vi "7.vi"   [LabVIEW 2020]
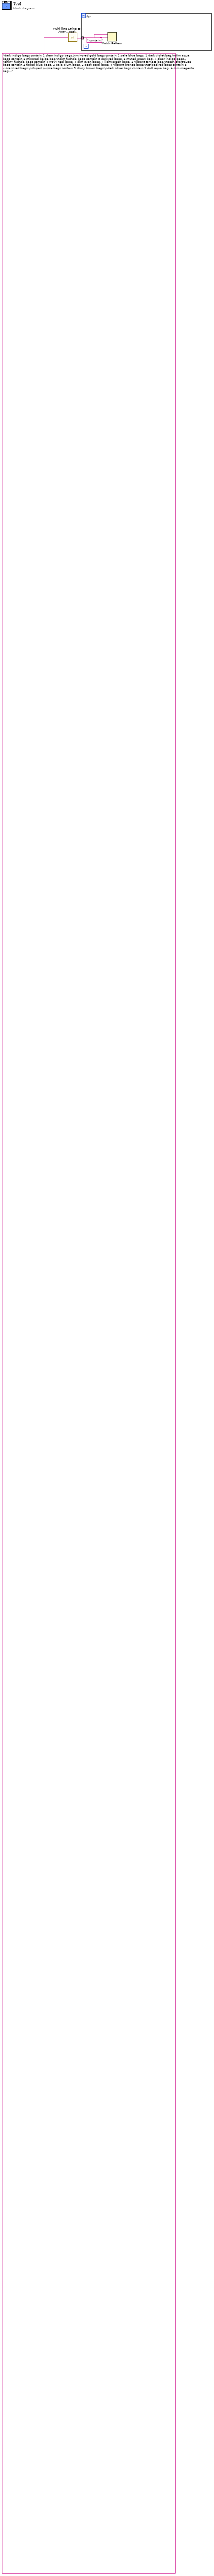
[diagram p0: block diagram]
diagram:
  n1 = call <userlib>:"Multi-line String to Array__ogtk.vi"("string"="dark indigo bags contain 2 clear indigo bags.\nmirrored gold bags contain 2 pale blue bags, 1 dark violet bag.\ndim aqua bags contain 1 mirrored beige bag.\ndim fuchsia bags contain 5 dark red bags, 1 muted green bag, 4 clear indigo bags.\nshiny fuchsia bags contain 4 wavy teal bags, 4 dim cyan bags, 4 light green bags, 1 vibrant tomato bag.\nposh chartreuse bags contain 2 faded blue bags, 2 pale plum bags, 2 posh coral bags, 4 vibrant bronze bags.\nstriped red bags contain 3 vibrant red bags.\nstriped purple bags contain 5 shiny brown bags.\ndark silver bags contain 1 dull aqua bag, 4 dim magenta bags.\ndark chartreuse bags contain 2 plaid black bags, 4 light bronze bags, 5 dotted cyan bags.\nshiny turquoise bags contain 1 shiny brown bag.\nshiny crimson bags contain no other bags.\nclear purple bags contain 4 bright red bags.\ndim white bags contain 4 posh violet bags, 2 light orange bags.\nplaid lime bags contain 4 muted silver bags, 2 vibrant tan bags.\nclear fuchsia bags contain 3 muted purple bags, 4 striped coral bags.\ndim plum bags contain 4 posh purple bags, 2 faded tomato bags, 1 mirrored magenta bag, 3 dull lime bags.\ndull white bags contain 4 light silver bags, 5 drab purple bags, 2 wavy orange bags, 1 striped coral bag.\ndull tomato bags contain 3 clear cyan bags, 5 dark turquoise bags, 4 light orange bags, 3 vibrant red bags.\nplaid tan bags contain 5 faded brown bags, 5 bright bronze bags.\nmirrored fuchsia bags contain 5 shiny brown bags, 3 dim magenta bags.\nwavy aqua bags contain 2 light beige bags, 3 vibrant white bags, 2 vibrant gold bags, 5 shiny tomato bags.\nclear white bags contain 3 dim maroon bags, 4 vibrant brown bags, 1 dim chartreuse bag.\nmuted yellow bags contain 3 shiny crimson bags, 4 posh purple bags, 2 dim plum bags, 3 shiny tomato bags.\nfaded cyan bags contain 5 mirrored crimson bags.\nposh violet bags contain 3 dim lavender bags, 3 vibrant teal bags.\nmirrored magenta bags contain 1 posh brown bag, 4 shiny teal bags, 2 shiny crimson bags.\nmirrored purple bags contain 2 clear aqua bags.\nwavy salmon bags contain 1 dull aqua bag, 1 dark silver bag.\nplaid purple bags contain 2 clear aqua bags, 5 pale brown bags, 3 bright chartreuse bags.\nposh teal bags contain 1 pale turquoise bag, 3 drab cyan bags.\npale tomato bags contain 2 dark beige bags.\nmuted plum bags contain 5 dotted gold bags, 5 shiny plum bags, 4 dull teal bags.\nwavy red bags contain 3 clear turquoise bags, 4 shiny chartreuse bags, 4 dotted maroon bags.\nwavy tomato bags contain 4 dark magenta bags, 1 faded bronze bag.\nshiny green bags contain 3 bright black bags, 2 clear turquoise bags.\nplaid turquoise bags contain 4 bright maroon bags.\nvibrant silver bags contain 5 bright chartreuse bags, 2 posh white bags, 3 drab tomato bags.\nposh olive bags contain 3 vibrant purple bags, 3 shiny crimson bags, 5 faded chartreuse bags.\nclear bronze bags contain 5 dark magenta bags.\nwavy teal bags contain 1 dim plum bag, 1 pale aqua bag, 2 posh purple bags, 2 pale orange bags.\nmuted beige bags contain 5 dotted brown bags, 4 mirrored green bags, 2 plaid blue bags.\nshiny maroon bags contain 2 pale green bags.\nwavy purple bags contain 5 dark bronze bags.\nvibrant cyan bags contain 2 drab blue bags, 5 pale brown bags, 1 mirrored magenta bag, 4 pale orange bags.\nwavy gray bags contain 5 pale crimson bags, 5 light aqua bags, 4 muted red bags.\nclear tomato bags contain 4 dark coral bags.\nshiny red bags contain 4 shiny tan bags, 4 pale cyan bags.\nmuted brown bags contain 5 dull olive bags, 2 pale silver bags, 5 faded plum bags.\nshiny violet bags contain 4 wavy teal bags.\nposh white bags contain 4 light fuchsia bags, 1 posh purple bag, 4 posh green bags.\ndim maroon bags contain 5 dim gold bags, 1 clear black bag.\ndull orange bags contain 1 clear teal bag, 3 dull gray bags.\nposh fuchsia bags contain 1 faded gold bag, 4 light bronze bags.\ndim bronze bags contain 1 bright fuchsia bag.\ndull salmon bags contain 5 muted tomato bags, 3 dull olive bags, 4 dark brown bags.\nposh yellow bags contain 5 dull indigo bags, 1 dotted green bag, 3 shiny chartreuse bags.\nmuted bronze bags contain 4 pale brown bags.\nwavy plum bags contain 4 shiny teal bags, 4 vibrant crimson bags.\ndark maroon bags contain 2 clear maroon bags, 3 light crimson bags.\nposh gray bags contain 2 drab maroon bags, 3 dotted aqua bags.\npale maroon bags contain 2 vibrant turquoise bags, 2 wavy tan bags, 5 clear orange bags, 2 clear beige bags.\nmirrored crimson bags contain 3 dark cyan bags, 3 dark silver bags.\nshiny bronze bags contain 3 drab tomato bags, 3 vibrant tan bags.\npale teal bags contain 4 clear brown bags, 4 vibrant gray bags, 3 bright plum bags, 4 dull olive bags.\nplaid maroon bags contain 1 mirrored blue bag, 4 bright chartreuse bags.\nplaid blue bags contain 4 light lime bags.\ndotted brown bags contain 5 shiny violet bags, 2 shiny lavender bags, 1 striped crimson bag.\npale purple bags contain 2 clear tomato bags, 5 vibrant orange bags, 5 dark green bags, 1 vibrant silver bag.\nclear lavender bags contain 1 wavy cyan bag, 5 dotted crimson bags, 5 dark bronze bags, 3 light bronze bags.\nlight cyan bags contain 5 light lime bags, 1 mirrored teal bag.\ndull blue bags contain 3 clear lime bags, 1 light turquoise bag, 1 shiny gray bag.\nfaded gray bags contain 2 faded crimson bags, 1 pale red bag, 3 striped bronze bags.\ndrab maroon bags contain 2 bright coral bags.\nplaid gold bags contain 2 shiny gold bags, 1 wavy fuchsia bag, 2 dull aqua bags, 4 mirrored indigo bags.\nmirrored orange bags contain 3 muted coral bags.\ndull yellow bags contain 1 drab maroon bag, 4 posh purple bags, 5 plaid cyan bags, 4 vibrant cyan bags.\nplaid aqua bags contain 2 bright silver bags, 2 posh blue bags, 3 drab olive bags, 2 mirrored fuchsia bags.\nshiny olive bags contain 3 dim tan bags, 1 dark gray bag, 4 mirrored brown bags, 5 mirrored magenta bags.\nwavy bronze bags contain 4 mirrored gray bags, 1 light lavender bag, 4 dull yellow bags.\ndotted orange bags contain 1 plaid teal bag, 5 pale silver bags, 1 drab bronze bag.\ndull magenta bags contain 1 muted violet bag, 2 muted black bags.\ndrab indigo bags contain 3 pale blue bags, 1 muted aqua bag, 3 bright fuchsia bags, 1 striped white bag.\nfaded turquoise bags contain 1 pale lavender bag, 1 shiny indigo bag.\nshiny lavender bags contain 2 faded bronze bags, 3 clear green bags, 5 dim turquoise bags, 5 striped olive bags.\nfaded yellow bags contain 1 faded chartreuse bag.\nvibrant gray bags contain 3 clear gold bags, 1 dotted coral bag, 4 light lime bags, 2 light lavender bags.\nbright aqua bags contain 2 faded chartreuse bags.\nbright yellow bags contain 4 dark blue bags.\nmirrored tomato bags contain 2 posh blue bags.\nshiny orange bags contain 3 striped black bags.\nbright tan bags contain 3 dim gold bags.\nlight fuchsia bags contain 4 dotted bronze bags, 2 posh purple bags.\nstriped coral bags contain 2 mirrored fuchsia bags, 4 faded chartreuse bags, 3 dull brown bags.\nbright cyan bags contain 3 mirrored lime bags, 2 posh purple bags, 3 light plum bags, 3 striped brown bags.\npale violet bags contain 3 wavy cyan bags.\nbright lavender bags contain 2 shiny crimson bags, 1 plaid magenta bag, 4 dark turquoise bags.\nwavy maroon bags contain 4 dull lavender bags, 2 dim turquoise bags, 2 light green bags, 1 clear lime bag.\ndrab tomato bags contain 1 light crimson bag, 5 faded gold bags, 5 drab cyan bags.\ndotted magenta bags contain 1 dotted beige bag.\nclear green bags contain 4 posh purple bags.\nshiny teal bags contain 2 pale turquoise bags.\nclear salmon bags contain 3 clear aqua bags.\ndark gold bags contain 1 pale tan bag.\nmirrored gray bags contain 1 muted purple bag.\nvibrant indigo bags contain 3 muted coral bags, 5 shiny gray bags, 1 dark yellow bag.\npale olive bags contain 2 posh white bags, 3 dull white bags, 5 light silver bags.\nbright bronze bags contain 3 dull yellow bags.\ndark yellow bags contain 1 bright black bag, 1 clear teal bag.\ndim cyan bags contain 4 wavy crimson bags, 4 muted green bags.\nshiny blue bags contain 1 pale beige bag, 1 plaid magenta bag, 1 dark magenta bag, 3 dim tomato bags.\npale green bags contain 5 dotted crimson bags, 5 posh purple bags, 4 pale aqua bags, 2 faded tomato bags.\nfaded coral bags contain 1 striped maroon bag, 5 drab salmon bags, 5 muted orange bags, 1 dark blue bag.\nlight beige bags contain 3 light red bags, 1 mirrored red bag, 3 drab salmon bags, 2 wavy teal bags.\nwavy yellow bags contain 2 clear coral bags, 2 pale turquoise bags.\ndim lavender bags contain 2 dull silver bags, 3 dull gray bags, 2 wavy crimson bags.\ndotted white bags contain 1 posh turquoise bag, 3 faded gold bags, 1 mirrored beige bag.\ndotted red bags contain 2 plaid gray bags.\nlight black bags contain 3 faded chartreuse bags, 4 dark yellow bags, 5 plaid cyan bags.\nvibrant black bags contain 2 faded fuchsia bags, 3 vibrant bronze bags, 3 dark brown bags, 5 bright purple bags.\nplaid olive bags contain 2 faded gray bags, 1 wavy purple bag.\npale plum bags contain 3 pale tan bags, 1 posh coral bag, 2 dim fuchsia bags.\nvibrant violet bags contain 1 clear coral bag.\nmirrored indigo bags contain 1 faded violet bag.\nposh lime bags contain 3 faded gray bags, 4 dim indigo bags, 1 wavy olive bag, 5 bright violet bags.\npale bronze bags contain 5 plaid gold bags.\nshiny purple bags contain 3 dark silver bags, 5 dark aqua bags, 5 mirrored indigo bags, 3 plaid teal bags.\nmuted turquoise bags contain 4 clear teal bags.\nlight turquoise bags contain 2 muted coral bags, 2 clear beige bags, 3 clear maroon bags.\nvibrant purple bags contain 4 dull aqua bags, 1 light crimson bag.\ndotted yellow bags contain 2 wavy yellow bags.\nbright salmon bags contain 5 striped coral bags, 4 dim red bags, 3 faded tan bags.\ndrab tan bags contain 2 clear yellow bags.\nplaid violet bags contain 2 pale plum bags, 3 dim lavender bags, 5 clear tan bags.\ndull tan bags contain 1 dotted aqua bag.\ndotted blue bags contain 4 vibrant maroon bags, 4 drab tomato bags, 5 light bronze bags, 1 posh bronze bag.\nlight silver bags contain 5 vibrant purple bags.\nmuted blue bags contain 4 bright coral bags, 3 faded blue bags, 5 dull lime bags, 5 pale brown bags.\ndotted lime bags contain 3 light aqua bags, 4 dull brown bags.\ndotted aqua bags contain 1 mirrored fuchsia bag, 5 wavy cyan bags, 3 wavy tan bags.\nfaded lavender bags contain 4 shiny chartreuse bags, 4 faded violet bags, 2 striped tan bags.\nbright violet bags contain 1 shiny gold bag, 5 pale beige bags, 2 pale orange bags, 3 wavy crimson bags.\nstriped turquoise bags contain 3 drab blue bags.\ndim black bags contain 2 muted coral bags, 2 pale plum bags, 2 shiny teal bags.\nstriped violet bags contain 5 mirrored white bags, 2 striped coral bags.\npale gray bags contain 4 faded chartreuse bags, 2 vibrant aqua bags.\ndrab cyan bags contain 5 bright fuchsia bags.\nwavy olive bags contain 3 striped beige bags.\nfaded aqua bags contain 4 vibrant teal bags, 1 dark olive bag, 1 bright crimson bag, 1 plaid indigo bag.\nwavy blue bags contain 4 clear maroon bags, 4 dim cyan bags, 2 mirrored gray bags.\nclear magenta bags contain 3 vibrant purple bags, 4 dotted maroon bags, 1 plaid green bag, 5 drab green bags.\nfaded olive bags contain 5 striped turquoise bags.\nvibrant olive bags contain 2 shiny teal bags, 4 shiny maroon bags, 5 clear tomato bags.\nmuted red bags contain 3 dim magenta bags, 1 shiny teal bag.\nbright indigo bags contain 5 muted red bags.\nfaded lime bags contain 5 posh maroon bags, 2 pale indigo bags, 2 posh turquoise bags, 5 dim indigo bags.\nplaid fuchsia bags contain 2 dim fuchsia bags, 3 light aqua bags.\nposh bronze bags contain 4 dull aqua bags.\nstriped green bags contain 1 dotted lime bag.\nfaded maroon bags contain 3 mirrored turquoise bags, 4 dark orange bags.\ndim turquoise bags contain 2 drab cyan bags, 2 clear lime bags, 2 dim salmon bags.\nbright gold bags contain 2 mirrored blue bags, 2 vibrant purple bags, 5 drab purple bags.\nlight red bags contain 1 drab fuchsia bag, 3 drab maroon bags, 5 dim plum bags, 5 pale red bags.\nvibrant lime bags contain 3 dull chartreuse bags, 4 pale crimson bags, 5 dark orange bags, 3 vibrant purple bags.\npale magenta bags contain 2 vibrant purple bags, 4 wavy olive bags.\ndrab turquoise bags contain 5 dotted crimson bags.\nposh beige bags contain 5 dark gray bags, 2 striped maroon bags, 3 muted red bags.\nwavy gold bags contain 2 dull lavender bags, 1 dotted red bag, 1 drab tomato bag, 4 dark gray bags.\nclear tan bags contain 5 dull gray bags, 2 wavy maroon bags, 2 pale red bags.\nwavy green bags contain 5 pale magenta bags, 2 vibrant coral bags, 2 bright turquoise bags.\nmirrored lavender bags contain 5 dotted beige bags.\nclear beige bags contain 2 muted purple bags.\nclear gray bags contain 5 shiny green bags, 3 plaid gold bags, 4 vibrant indigo bags, 1 pale brown bag.\nmirrored lime bags contain 1 muted gray bag, 1 striped red bag, 5 plaid brown bags, 1 plaid black bag.\nclear olive bags contain 1 posh olive bag, 1 striped bronze bag.\nwavy lavender bags contain 3 mirrored green bags, 3 bright coral bags.\nmuted green bags contain 4 pale orange bags.\nposh black bags contain 1 wavy bronze bag, 2 dim cyan bags.\nposh purple bags contain no other bags.\nwavy crimson bags contain 3 dim fuchsia bags, 5 dull chartreuse bags, 1 dark yellow bag.\nbright lime bags contain 2 pale crimson bags, 2 drab green bags, 3 dull orange bags.\nmirrored black bags contain 5 light beige bags, 1 striped olive bag, 2 plaid purple bags, 3 vibrant tan bags.\ndull turquoise bags contain 5 striped violet bags, 3 striped lime bags, 4 pale black bags, 3 drab brown bags.\nstriped yellow bags contain 2 dark crimson bags, 1 clear fuchsia bag.\ndrab orange bags contain 3 shiny blue bags, 2 clear green bags, 2 muted plum bags.\nlight coral bags contain 3 mirrored fuchsia bags, 1 shiny tomato bag, 2 dull aqua bags, 2 muted yellow bags.\nposh silver bags contain 1 light coral bag.\nlight tomato bags contain 1 faded silver bag.\ndark turquoise bags contain 3 dull yellow bags, 4 posh turquoise bags.\ndotted olive bags contain 2 clear bronze bags.\nfaded beige bags contain 5 posh teal bags, 2 drab beige bags, 3 plaid lavender bags, 4 drab purple bags.\ndrab lavender bags contain 4 faded gray bags, 2 pale blue bags, 4 faded gold bags, 3 dark silver bags.\nfaded salmon bags contain 5 light lavender bags.\ndrab crimson bags contain 3 drab aqua bags, 4 striped yellow bags, 2 shiny fuchsia bags, 4 dark olive bags.\nclear brown bags contain 1 striped coral bag, 2 shiny gold bags.\nwavy black bags contain 3 dull orange bags, 3 faded salmon bags, 2 plaid white bags.\nfaded brown bags contain 2 plaid cyan bags, 5 light lavender bags, 3 bright coral bags, 2 drab maroon bags.\nvibrant yellow bags contain 4 striped bronze bags.\nposh aqua bags contain 4 light crimson bags, 1 dark red bag, 4 bright lavender bags, 4 striped beige bags.\npale cyan bags contain 1 dark olive bag, 2 pale orange bags, 1 vibrant white bag.\nmuted white bags contain 1 light brown bag.\nbright fuchsia bags contain 2 posh brown bags, 5 clear coral bags, 1 dim plum bag.\nmirrored aqua bags contain 3 light fuchsia bags, 3 bright aqua bags, 2 light aqua bags.\nwavy coral bags contain 2 muted yellow bags, 3 drab silver bags, 5 dark silver bags.\nmuted fuchsia bags contain 1 plaid black bag, 5 shiny yellow bags.\ndim green bags contain 4 wavy aqua bags, 2 light cyan bags, 1 shiny gray bag.\ndrab black bags contain 2 dotted maroon bags, 5 clear maroon bags, 3 mirrored coral bags, 1 dim salmon bag.\nshiny coral bags contain 4 light plum bags, 4 mirrored chartreuse bags, 3 wavy white bags.\nposh indigo bags contain 2 dark cyan bags, 5 pale brown bags, 1 dull blue bag, 3 striped red bags.\npale brown bags contain 4 dull red bags, 4 shiny teal bags, 4 shiny crimson bags, 2 bright fuchsia bags.\nplaid coral bags contain 1 dim maroon bag, 4 clear plum bags, 5 dark green bags, 4 shiny purple bags.\nshiny gold bags contain 1 pale aqua bag, 3 dark cyan bags, 5 vibrant purple bags, 2 drab blue bags.\nplaid brown bags contain 1 wavy crimson bag.\nmuted teal bags contain 2 drab turquoise bags, 2 clear tan bags, 4 shiny violet bags, 1 vibrant tan bag.\ndrab blue bags contain 2 bright fuchsia bags, 2 clear coral bags.\nlight olive bags contain 2 faded purple bags, 4 striped bronze bags.\ndrab yellow bags contain 5 shiny maroon bags, 4 clear teal bags, 5 wavy white bags.\nclear blue bags contain 5 drab maroon bags, 2 shiny gold bags, 3 pale red bags, 3 dotted gold bags.\nwavy brown bags contain 2 pale beige bags, 5 light yellow bags, 4 striped aqua bags, 3 wavy yellow bags.\ndotted purple bags contain 2 dark teal bags, 5 posh brown bags, 4 plaid fuchsia bags, 2 posh silver bags.\nmirrored turquoise bags contain 3 dim tan bags.\ndotted cyan bags contain 3 shiny lavender bags, 5 clear aqua bags.\nstriped olive bags contain 4 dark cyan bags, 3 dim plum bags.\nfaded fuchsia bags contain 1 shiny indigo bag, 2 dull gold bags, 4 mirrored salmon bags.\npale gold bags contain 4 clear gold bags, 3 bright lime bags.\ndull olive bags contain 4 striped chartreuse bags.\nshiny tomato bags contain 4 shiny teal bags.\nstriped salmon bags contain 5 faded lavender bags, 1 dim aqua bag.\npale salmon bags contain 2 dim orange bags.\ndim salmon bags contain 3 posh purple bags, 5 mirrored brown bags.\nmuted coral bags contain 4 light green bags, 3 striped turquoise bags, 2 plaid silver bags, 5 vibrant maroon bags.\ndull bronze bags contain 2 dim magenta bags, 1 faded lavender bag.\ndrab gray bags contain 1 mirrored indigo bag, 1 pale crimson bag, 3 plaid teal bags.\nmuted chartreuse bags contain 5 light coral bags, 5 vibrant turquoise bags, 3 dark cyan bags, 5 bright orange bags.\nmirrored green bags contain 2 bright purple bags, 4 posh bronze bags, 1 shiny violet bag, 5 clear teal bags.\nbright orange bags contain 1 dull gray bag.\ndim coral bags contain 1 posh salmon bag, 2 striped salmon bags, 3 striped chartreuse bags.\nclear turquoise bags contain 3 wavy salmon bags, 1 clear blue bag, 1 drab tan bag.\nbright teal bags contain 1 faded tan bag, 5 striped teal bags, 3 light lavender bags, 2 dark olive bags.\nshiny chartreuse bags contain 2 dull blue bags, 5 drab turquoise bags, 4 light aqua bags.\nfaded tan bags contain 4 drab purple bags.\nplaid magenta bags contain 5 drab cyan bags, 4 muted aqua bags.\nmuted purple bags contain no other bags.\nvibrant green bags contain 5 striped crimson bags, 5 clear beige bags, 3 drab yellow bags.\nvibrant salmon bags contain 4 clear red bags, 5 wavy salmon bags.\nvibrant tomato bags contain 3 light plum bags, 1 posh white bag, 2 wavy magenta bags.\nwavy turquoise bags contain 5 dotted gold bags, 2 light gray bags, 4 drab tomato bags, 5 wavy aqua bags.\ndim olive bags contain 3 light magenta bags, 1 dotted lime bag, 4 dotted crimson bags, 3 light salmon bags.\nplaid lavender bags contain 2 dark turquoise bags, 5 striped turquoise bags, 4 wavy olive bags.\ndark green bags contain 3 dotted gold bags.\nfaded purple bags contain 5 clear coral bags, 3 mirrored green bags, 5 drab coral bags, 3 bright purple bags.\ndotted crimson bags contain 2 wavy teal bags, 5 light green bags, 5 muted purple bags, 1 plaid silver bag.\nmirrored coral bags contain 5 striped turquoise bags, 1 faded purple bag, 1 shiny cyan bag.\nmirrored cyan bags contain 1 mirrored chartreuse bag, 5 wavy magenta bags.\nshiny black bags contain 2 drab magenta bags, 2 plaid bronze bags.\ndark teal bags contain 3 dark white bags, 1 muted chartreuse bag, 3 dotted salmon bags, 4 posh aqua bags.\ndull teal bags contain 2 bright chartreuse bags, 3 light black bags.\nmirrored red bags contain 2 dotted crimson bags, 2 drab cyan bags.\nstriped brown bags contain 2 pale red bags, 5 light gray bags.\nposh magenta bags contain 4 posh green bags, 4 dotted bronze bags, 5 dim tan bags.\npale lime bags contain 5 shiny blue bags.\nplaid indigo bags contain 3 shiny maroon bags, 1 dark yellow bag, 4 dull gold bags.\nlight green bags contain 2 dull brown bags, 5 bright coral bags.\nmuted olive bags contain 3 dotted bronze bags, 1 shiny coral bag, 3 dotted aqua bags, 2 faded blue bags.\nstriped lime bags contain 2 faded salmon bags, 2 pale white bags, 1 plaid salmon bag, 1 dark coral bag.\nclear red bags contain 3 dark orange bags, 5 faded magenta bags, 4 dark lime bags.\nfaded bronze bags contain 4 light lavender bags.\ndotted plum bags contain 1 faded tan bag, 3 pale aqua bags, 2 dull gray bags, 4 plaid purple bags.\nplaid salmon bags contain 5 light lime bags, 1 posh bronze bag, 5 wavy magenta bags, 1 dark green bag.\ndull plum bags contain 4 mirrored purple bags.\nlight indigo bags contain 3 dark silver bags, 1 bright lime bag.\npale red bags contain 5 posh purple bags.\nwavy chartreuse bags contain 1 light coral bag.\ndull lavender bags contain 5 plaid purple bags, 4 faded orange bags.\nvibrant orange bags contain 2 drab violet bags.\nlight gold bags contain 3 plaid salmon bags.\nfaded teal bags contain 1 dotted maroon bag.\nlight chartreuse bags contain 3 dotted yellow bags, 1 clear yellow bag, 3 shiny teal bags, 4 plaid lime bags.\nfaded white bags contain 5 drab turquoise bags, 1 dark violet bag.\nlight lavender bags contain 1 vibrant magenta bag, 1 pale brown bag.\nlight crimson bags contain 5 dull red bags.\nmirrored silver bags contain 2 bright turquoise bags.\nfaded green bags contain 5 dark lime bags, 5 dim crimson bags, 4 dark silver bags, 1 dotted white bag.\nvibrant chartreuse bags contain 5 wavy gray bags, 5 bright silver bags, 1 dull indigo bag.\nclear chartreuse bags contain 5 light brown bags, 2 dim violet bags, 4 faded orange bags.\ndotted violet bags contain 4 dark white bags, 1 muted brown bag, 4 faded cyan bags, 5 striped gray bags.\ndotted green bags contain 5 bright silver bags, 4 drab lime bags.\nlight bronze bags contain 3 dotted gold bags.\nvibrant tan bags contain 2 dull chartreuse bags, 5 clear gold bags, 1 bright orange bag, 2 dotted gold bags.\nfaded gold bags contain 4 shiny gold bags, 1 dark red bag, 2 dotted bronze bags, 1 muted red bag.\nplaid green bags contain 4 light gray bags, 1 striped bronze bag.\nclear yellow bags contain 4 drab blue bags.\nmirrored yellow bags contain 3 vibrant tan bags, 2 light crimson bags, 1 light lime bag, 5 bright teal bags.\ndotted beige bags contain 2 pale beige bags, 3 light lime bags, 3 drab cyan bags, 3 plaid green bags.\npale chartreuse bags contain 1 striped brown bag, 2 faded gold bags.\nwavy white bags contain 4 dotted gold bags, 5 striped turquoise bags, 1 mirrored chartreuse bag.\nmuted tomato bags contain 5 dark magenta bags.\ndark lavender bags contain 4 pale indigo bags, 5 shiny cyan bags.\npale black bags contain 3 clear tomato bags, 3 vibrant gray bags.\ndim orange bags contain 5 dark olive bags, 1 vibrant silver bag, 3 plaid brown bags, 1 dull red bag.\nbright plum bags contain 5 striped tomato bags, 2 dotted beige bags.\nposh tomato bags contain 5 faded tomato bags.\nvibrant maroon bags contain 5 dark orange bags.\ndim tan bags contain 5 muted yellow bags.\ndotted tan bags contain 4 dark lime bags.\nplaid red bags contain 2 posh beige bags, 3 wavy tan bags, 1 muted silver bag.\nfaded black bags contain 1 clear lavender bag, 4 dotted lime bags, 3 mirrored crimson bags, 2 faded gray bags.\nmirrored tan bags contain 2 vibrant white bags, 5 mirrored beige bags, 4 wavy turquoise bags, 4 striped green bags.\ndull violet bags contain 5 bright teal bags.\nstriped maroon bags contain 2 dull brown bags.\ndull green bags contain 4 dim yellow bags, 3 mirrored silver bags, 5 muted chartreuse bags.\ndull gray bags contain 3 vibrant purple bags, 3 striped turquoise bags, 5 wavy cyan bags.\nposh salmon bags contain 4 light green bags, 4 dull blue bags.\ndark tan bags contain 5 muted bronze bags, 5 clear lime bags, 5 vibrant gray bags.\ndark purple bags contain 1 clear cyan bag, 3 vibrant tan bags, 5 light magenta bags, 1 dark blue bag.\nplaid teal bags contain 1 wavy purple bag, 4 mirrored crimson bags.\nposh brown bags contain no other bags.\npale orange bags contain no other bags.\nposh plum bags contain 3 light bronze bags, 3 bright coral bags, 3 shiny yellow bags, 3 dark yellow bags.\nbright olive bags contain 2 light silver bags.\nposh red bags contain 4 dark turquoise bags, 1 plaid cyan bag, 3 dotted aqua bags.\nmuted violet bags contain 3 pale green bags, 5 dull red bags.\nplaid crimson bags contain 3 clear silver bags.\ndotted gray bags contain 1 muted white bag.\ndull brown bags contain 1 dull aqua bag, 4 bright coral bags, 5 shiny violet bags, 1 light coral bag.\npale silver bags contain 3 mirrored brown bags, 2 dark brown bags, 2 vibrant indigo bags.\nvibrant coral bags contain 2 pale red bags, 3 bright teal bags, 5 striped bronze bags, 1 bright silver bag.\ndark brown bags contain 1 pale brown bag, 1 drab beige bag, 4 mirrored chartreuse bags, 1 clear teal bag.\ndotted turquoise bags contain 4 wavy chartreuse bags, 2 faded violet bags.\nbright silver bags contain 3 dark silver bags, 5 clear aqua bags, 1 striped coral bag, 4 vibrant violet bags.\nplaid chartreuse bags contain 3 pale red bags, 4 wavy teal bags, 3 dark tomato bags.\nbright red bags contain 4 pale red bags.\npale beige bags contain 3 posh purple bags, 2 striped gold bags.\nvibrant plum bags contain 3 posh green bags, 5 plaid cyan bags, 4 light silver bags.\nbright white bags contain 3 dull gold bags, 5 striped turquoise bags, 2 bright tan bags.\ndark magenta bags contain 1 pale aqua bag, 5 faded bronze bags, 3 dark orange bags, 3 dim magenta bags.\nbright beige bags contain 4 clear white bags, 2 dotted plum bags, 2 light brown bags, 1 plaid gray bag.\nbright black bags contain 2 pale turquoise bags, 5 mirrored brown bags, 1 mirrored magenta bag, 4 dull lime bags.\nbright gray bags contain 3 mirrored red bags, 5 clear brown bags, 4 muted violet bags.\nmuted magenta bags contain 1 posh bronze bag, 5 mirrored brown bags, 1 clear crimson bag, 1 light lavender bag.\nlight teal bags contain 4 shiny tan bags.\ndark gray bags contain 4 dotted bronze bags, 2 pale red bags, 3 pale brown bags, 5 dim magenta bags.\nmuted black bags contain 5 light beige bags, 1 dark tomato bag, 3 striped coral bags, 3 vibrant maroon bags.\ndark red bags contain 5 muted red bags, 3 dull lime bags, 2 shiny tomato bags, 2 pale brown bags.\nbright brown bags contain 4 bright teal bags, 3 plaid green bags.\nplaid yellow bags contain 4 plaid bronze bags.\ndark cyan bags contain 2 dim plum bags, 4 shiny brown bags.\nfaded blue bags contain 4 faded yellow bags.\ndull maroon bags contain 3 mirrored purple bags, 2 faded silver bags, 5 pale silver bags.\nposh coral bags contain 5 dim gold bags.\nfaded chartreuse bags contain 2 clear coral bags, 5 dim gold bags.\nstriped silver bags contain 4 faded cyan bags, 5 wavy brown bags, 5 bright tan bags, 3 drab chartreuse bags.\nplaid gray bags contain 4 faded tomato bags, 4 dim cyan bags, 4 dotted maroon bags, 5 clear indigo bags.\nplaid white bags contain 4 dim magenta bags, 4 pale red bags.\ndark black bags contain 1 drab tan bag, 4 striped indigo bags.\nvibrant white bags contain 1 dull aqua bag, 3 dull red bags.\nmuted maroon bags contain 3 dim violet bags, 3 faded orange bags, 1 bright purple bag, 2 dull cyan bags.\npale indigo bags contain 3 faded plum bags, 3 clear tomato bags.\nclear teal bags contain 1 light coral bag, 5 faded bronze bags, 5 faded chartreuse bags, 2 striped olive bags.\nmuted tan bags contain 3 bright cyan bags.\nlight magenta bags contain 5 dark magenta bags, 3 striped brown bags.\ndark aqua bags contain 3 posh turquoise bags, 4 pale fuchsia bags, 2 bright orange bags, 4 dim cyan bags.\nbright tomato bags contain 5 wavy bronze bags, 4 clear magenta bags, 4 shiny fuchsia bags.\ndark salmon bags contain 4 pale indigo bags, 4 wavy magenta bags.\ndim blue bags contain 4 pale magenta bags, 2 muted tomato bags.\ndark blue bags contain 4 shiny tomato bags.\ndrab aqua bags contain 5 clear cyan bags, 1 dotted orange bag.\nplaid tomato bags contain 2 clear red bags, 2 dark tomato bags, 2 bright gold bags.\nvibrant crimson bags contain 3 dull blue bags.\nlight yellow bags contain 2 striped black bags, 2 shiny brown bags, 5 clear black bags.\npale white bags contain 1 posh plum bag.\ndull gold bags contain 5 wavy crimson bags, 5 pale aqua bags, 5 mirrored cyan bags, 2 drab tomato bags.\nstriped gray bags contain 5 shiny tomato bags, 3 mirrored brown bags, 1 posh brown bag.\ndrab salmon bags contain 5 vibrant yellow bags.\nlight purple bags contain 1 shiny turquoise bag.\nstriped lavender bags contain 4 mirrored gold bags, 3 vibrant brown bags, 3 wavy bronze bags, 2 pale black bags.\nvibrant beige bags contain 2 light yellow bags.\nstriped magenta bags contain 4 light black bags.\nclear aqua bags contain 2 dark cyan bags, 1 faded orange bag, 3 mirrored gray bags, 2 dark tomato bags.\ndim teal bags contain 2 dark gray bags.\nstriped tomato bags contain 4 dark coral bags, 1 faded blue bag.\nstriped gold bags contain 4 bright coral bags, 1 shiny teal bag, 4 dark silver bags.\nlight maroon bags contain 4 dotted coral bags.\npale blue bags contain 2 striped coral bags, 1 vibrant white bag, 3 drab maroon bags.\nclear crimson bags contain 3 plaid chartreuse bags, 1 pale bronze bag.\ndim beige bags contain 5 drab tan bags.\npale turquoise bags contain no other bags.\ndotted salmon bags contain 2 clear magenta bags, 4 pale silver bags.\nposh orange bags contain 3 dull aqua bags, 3 vibrant gray bags, 4 dull olive bags, 1 mirrored magenta bag.\ndark tomato bags contain 3 shiny lavender bags, 2 drab beige bags, 3 dark cyan bags.\nshiny aqua bags contain 3 light maroon bags, 4 muted turquoise bags, 2 vibrant magenta bags.\nbright purple bags contain 3 light silver bags, 3 mirrored magenta bags.\nshiny lime bags contain 3 dark olive bags, 1 striped chartreuse bag, 1 muted green bag.\nbright crimson bags contain 2 muted indigo bags.\nclear silver bags contain 3 mirrored red bags.\nbright coral bags contain 1 dim gold bag, 2 clear green bags, 3 dark cyan bags.\npale crimson bags contain 4 shiny teal bags, 5 drab maroon bags, 1 pale brown bag.\nwavy silver bags contain 2 dotted cyan bags, 1 vibrant silver bag, 2 light turquoise bags, 3 light salmon bags.\nmuted salmon bags contain 1 shiny bronze bag, 5 faded salmon bags, 4 muted black bags, 1 muted coral bag.\ndrab teal bags contain 2 vibrant violet bags, 4 vibrant orange bags.\nmirrored blue bags contain 3 mirrored fuchsia bags.\nmirrored white bags contain 4 striped brown bags, 5 mirrored cyan bags.\ndull coral bags contain 2 bright magenta bags, 5 clear tan bags.\ndull aqua bags contain 3 dim magenta bags, 2 light lavender bags.\nfaded crimson bags contain 4 striped maroon bags, 4 dull lime bags, 5 vibrant magenta bags.\nlight blue bags contain 1 plaid gold bag, 5 plaid white bags, 1 plaid black bag.\npale tan bags contain 3 posh green bags, 1 dim fuchsia bag, 5 vibrant yellow bags.\nvibrant blue bags contain 4 pale gold bags, 1 clear magenta bag.\nvibrant red bags contain 1 plaid cyan bag, 2 dim tan bags, 1 muted red bag.\nstriped cyan bags contain 5 plaid blue bags, 3 faded lavender bags.\ndull silver bags contain 2 dark bronze bags, 5 pale orange bags.\nstriped bronze bags contain 1 shiny tomato bag, 4 muted yellow bags, 4 striped turquoise bags.\nlight aqua bags contain 5 shiny violet bags.\ndrab white bags contain 5 faded gold bags, 1 striped tomato bag, 1 plaid salmon bag.\nclear lime bags contain 4 mirrored brown bags, 2 light lavender bags, 1 light coral bag.\nshiny tan bags contain 4 bright fuchsia bags, 1 dark orange bag, 1 dull lime bag.\nbright turquoise bags contain 1 dim salmon bag, 3 light green bags, 3 shiny crimson bags, 2 wavy cyan bags.\nposh lavender bags contain 1 bright bronze bag, 2 dull lavender bags, 1 vibrant purple bag, 5 shiny violet bags.\nwavy indigo bags contain 2 striped violet bags, 1 mirrored red bag, 1 muted turquoise bag.\ndull cyan bags contain 5 vibrant yellow bags, 2 wavy salmon bags, 2 striped olive bags, 5 vibrant turquoise bags.\nposh maroon bags contain 2 clear bronze bags, 3 vibrant tan bags.\nfaded violet bags contain 4 shiny olive bags, 3 posh magenta bags.\nstriped blue bags contain 4 dull tomato bags, 3 bright plum bags.\nmirrored teal bags contain 4 dark crimson bags, 5 dotted coral bags, 2 clear indigo bags, 5 faded salmon bags.\nbright magenta bags contain 4 clear turquoise bags, 5 dim turquoise bags.\nvibrant magenta bags contain 5 mirrored magenta bags, 2 clear green bags.\nclear cyan bags contain 4 pale turquoise bags, 3 wavy maroon bags.\nstriped beige bags contain 5 mirrored magenta bags, 4 clear fuchsia bags.\nlight white bags contain 4 pale brown bags, 3 vibrant plum bags.\nshiny silver bags contain 5 striped gray bags, 3 drab silver bags, 3 shiny beige bags, 4 wavy salmon bags.\ndrab magenta bags contain 5 dark brown bags, 4 shiny fuchsia bags.\ndark white bags contain 5 posh fuchsia bags, 4 shiny turquoise bags, 1 vibrant cyan bag.\ndim red bags contain 1 bright tan bag.\nposh crimson bags contain 5 bright gray bags.\nplaid silver bags contain 4 muted purple bags, 5 faded gold bags.\ndull indigo bags contain 5 dim violet bags, 5 light maroon bags.\ndotted fuchsia bags contain 4 pale yellow bags, 5 dim gold bags, 2 bright fuchsia bags.\nlight lime bags contain 4 striped aqua bags, 4 shiny tan bags, 2 striped bronze bags, 4 dotted lime bags.\ndark crimson bags contain 2 dim turquoise bags.\nplaid bronze bags contain 3 posh red bags, 4 mirrored silver bags, 2 drab tan bags.\ndark plum bags contain 1 pale coral bag, 4 clear cyan bags, 5 dim turquoise bags, 4 striped crimson bags.\nmirrored maroon bags contain 5 clear chartreuse bags, 2 pale purple bags, 5 clear fuchsia bags.\ndrab fuchsia bags contain 2 shiny olive bags, 5 wavy salmon bags, 5 drab lime bags.\nbright chartreuse bags contain 5 bright turquoise bags, 3 bright fuchsia bags.\ndim indigo bags contain 4 wavy chartreuse bags, 3 light coral bags, 1 clear fuchsia bag, 2 faded violet bags.\nvibrant brown bags contain 4 mirrored silver bags, 4 bright bronze bags, 3 plaid purple bags.\nstriped black bags contain 3 shiny fuchsia bags.\nwavy orange bags contain 3 clear maroon bags, 5 drab magenta bags.\nstriped indigo bags contain 4 striped teal bags, 5 dull lavender bags, 1 muted red bag, 3 wavy blue bags.\ndark bronze bags contain 3 clear beige bags, 4 drab cyan bags.\nstriped crimson bags contain 1 plaid cyan bag.\nlight salmon bags contain 5 pale yellow bags, 2 plaid purple bags, 4 dark indigo bags, 3 striped white bags.\ndotted indigo bags contain 3 mirrored magenta bags, 5 striped gold bags, 3 clear coral bags, 2 wavy olive bags.\nmuted gold bags contain 3 wavy violet bags, 1 wavy purple bag, 2 dim gold bags.\nclear orange bags contain 1 striped turquoise bag, 3 posh turquoise bags, 3 light plum bags, 3 pale crimson bags.\nfaded magenta bags contain 1 drab blue bag, 2 plaid green bags.\ndark orange bags contain 4 drab tomato bags, 4 mirrored brown bags, 1 mirrored fuchsia bag, 1 dim magenta bag.\npale fuchsia bags contain 1 clear lime bag.\ndotted teal bags contain 1 dull fuchsia bag.\ndrab silver bags contain 4 pale red bags, 4 clear chartreuse bags.\nclear gold bags contain 4 pale crimson bags.\ndotted bronze bags contain 4 mirrored brown bags, 2 dull red bags, 1 shiny tomato bag.\nshiny brown bags contain no other bags.\npale yellow bags contain 2 mirrored brown bags, 5 clear fuchsia bags.\ndull chartreuse bags contain 4 posh magenta bags, 3 mirrored magenta bags.\ndim silver bags contain 3 faded coral bags.\ndull purple bags contain 1 light blue bag, 5 dark fuchsia bags, 5 faded lavender bags, 3 posh maroon bags.\nlight violet bags contain 5 dim olive bags.\nwavy fuchsia bags contain 1 shiny olive bag, 4 drab cyan bags.\nmuted aqua bags contain 1 shiny teal bag, 1 dull lime bag, 5 faded tomato bags, 5 bright fuchsia bags.\nstriped orange bags contain 5 mirrored beige bags.\nfaded orange bags contain 2 wavy yellow bags, 2 bright fuchsia bags, 3 posh purple bags.\ndotted lavender bags contain 5 dark blue bags, 3 faded black bags, 4 bright indigo bags.\nwavy tan bags contain 3 plaid chartreuse bags, 1 clear gold bag.\nclear indigo bags contain 4 striped olive bags, 3 mirrored brown bags.\nlight plum bags contain 3 mirrored indigo bags.\nstriped tan bags contain 2 vibrant cyan bags, 4 dull lime bags, 2 dim indigo bags.\nplaid cyan bags contain 1 dim turquoise bag, 5 clear lime bags, 1 muted yellow bag, 3 shiny brown bags.\ndrab gold bags contain 1 pale red bag, 4 shiny purple bags.\ndrab violet bags contain 5 vibrant lime bags, 3 vibrant aqua bags.\ndim gold bags contain 5 dull lime bags, 3 bright fuchsia bags, 1 muted yellow bag.\nmuted cyan bags contain 1 mirrored black bag, 2 clear orange bags, 5 light crimson bags, 2 mirrored teal bags.\ndotted tomato bags contain 1 dotted bronze bag, 1 dark orange bag, 4 vibrant maroon bags, 5 drab tomato bags.\nstriped chartreuse bags contain 4 mirrored fuchsia bags, 5 dim magenta bags.\nmuted silver bags contain 1 vibrant turquoise bag, 1 clear teal bag, 3 bright black bags.\ndim purple bags contain 2 light gray bags, 2 dull aqua bags, 1 pale turquoise bag, 3 dim gold bags.\ndrab red bags contain 4 drab magenta bags.\nmuted indigo bags contain 4 light plum bags, 1 striped beige bag.\ndark olive bags contain 4 striped gold bags.\nclear violet bags contain 5 vibrant white bags, 1 wavy bronze bag, 3 light plum bags, 1 dark yellow bag.\nstriped aqua bags contain 3 dim salmon bags, 3 light aqua bags.\nbright maroon bags contain 4 shiny fuchsia bags, 5 faded tomato bags, 1 clear white bag, 4 wavy yellow bags.\ndark beige bags contain 4 faded blue bags, 4 vibrant bronze bags, 2 dark magenta bags.\nposh turquoise bags contain 4 pale red bags, 3 mirrored brown bags, 3 mirrored indigo bags, 3 striped gold bags.\ndrab purple bags contain 5 light green bags, 1 shiny gold bag, 2 striped turquoise bags, 5 mirrored beige bags.\nbright blue bags contain 5 dim indigo bags, 2 dotted crimson bags, 1 bright aqua bag, 5 clear silver bags.\nposh blue bags contain 2 shiny maroon bags, 3 striped bronze bags.\nwavy beige bags contain 1 dotted white bag, 3 striped aqua bags, 3 drab yellow bags.\ndotted chartreuse bags contain 5 dotted bronze bags.\nshiny gray bags contain 2 dim magenta bags.\nmirrored beige bags contain 3 clear coral bags, 3 dim salmon bags.\nfaded tomato bags contain 2 bright black bags, 5 shiny tomato bags, 3 mirrored brown bags, 5 dull lime bags.\ndrab brown bags contain 5 clear black bags.\nclear black bags contain 4 faded blue bags, 4 posh turquoise bags, 4 pale green bags, 4 faded crimson bags.\nvibrant aqua bags contain 2 faded bronze bags, 3 dull aqua bags, 1 clear beige bag, 2 light lavender bags.\ndrab green bags contain 3 drab blue bags, 2 pale red bags, 2 posh green bags.\nwavy cyan bags contain 4 faded blue bags, 2 faded chartreuse bags, 2 pale crimson bags.\nplaid orange bags contain 1 muted yellow bag, 5 dull chartreuse bags, 5 dull gray bags, 3 pale crimson bags.\ndark lime bags contain 4 clear brown bags, 1 drab fuchsia bag, 1 light aqua bag, 4 wavy tan bags.\ndark violet bags contain 3 vibrant lime bags, 3 clear fuchsia bags.\nplaid beige bags contain 2 dark teal bags, 2 posh indigo bags, 4 mirrored red bags, 3 vibrant gold bags.\nstriped fuchsia bags contain 1 dim tan bag, 4 dotted plum bags, 5 plaid olive bags.\npale aqua bags contain 4 shiny tomato bags, 3 bright black bags.\nshiny magenta bags contain 5 plaid blue bags, 2 pale maroon bags, 2 dim lavender bags.\ndotted black bags contain 2 shiny aqua bags, 2 dim crimson bags, 2 plaid red bags, 5 bright black bags.\nclear coral bags contain no other bags.\nshiny yellow bags contain 2 clear silver bags, 1 vibrant cyan bag, 3 striped crimson bags, 5 light aqua bags.\ndull beige bags contain 3 light green bags.\ndrab beige bags contain 4 bright black bags, 4 light silver bags, 4 light lavender bags.\nshiny salmon bags contain 2 light blue bags, 1 pale yellow bag.\npale lavender bags contain 2 shiny maroon bags, 5 posh tan bags.\nmuted crimson bags contain 1 clear aqua bag, 2 posh turquoise bags.\ndim gray bags contain 4 pale tomato bags, 2 dark chartreuse bags, 4 clear red bags.\nfaded silver bags contain 2 drab beige bags, 3 faded tomato bags, 4 dull gold bags, 2 mirrored magenta bags.\nlight gray bags contain 5 dark yellow bags.\ndotted gold bags contain 1 light plum bag, 2 faded tomato bags.\ndrab chartreuse bags contain 4 vibrant indigo bags.\ndim tomato bags contain 5 clear gold bags, 4 light gray bags, 4 shiny green bags, 5 faded yellow bags.\ndull fuchsia bags contain 3 vibrant cyan bags, 1 dim plum bag, 5 posh bronze bags, 1 shiny crimson bag.\nshiny cyan bags contain 5 striped red bags, 5 dim plum bags, 2 striped turquoise bags.\ndim yellow bags contain 1 dull chartreuse bag.\nwavy magenta bags contain 2 dull lime bags, 2 mirrored chartreuse bags, 2 faded bronze bags.\nposh tan bags contain 5 shiny tomato bags, 5 drab maroon bags, 5 vibrant maroon bags.\nvibrant gold bags contain 1 dark orange bag, 2 mirrored cyan bags, 1 vibrant cyan bag, 2 posh coral bags.\nvibrant fuchsia bags contain 2 vibrant violet bags.\nmuted orange bags contain 3 striped gold bags, 1 posh green bag, 3 vibrant purple bags.\nmirrored violet bags contain 4 clear chartreuse bags, 4 dotted yellow bags, 2 faded orange bags.\ndrab lime bags contain 1 mirrored magenta bag, 1 striped turquoise bag.\ndotted silver bags contain 2 dark cyan bags, 5 drab olive bags.\ndull crimson bags contain 3 clear yellow bags, 3 vibrant cyan bags, 1 bright turquoise bag.\nlight brown bags contain 4 shiny brown bags, 1 plaid fuchsia bag.\nvibrant teal bags contain 2 mirrored aqua bags, 5 plaid silver bags.\nvibrant turquoise bags contain 2 clear beige bags.\nvibrant lavender bags contain 2 shiny teal bags, 5 shiny blue bags, 2 dull gray bags, 1 muted crimson bag.\nbright green bags contain 1 dull silver bag, 1 dull red bag, 4 vibrant indigo bags, 2 clear coral bags.\nmirrored bronze bags contain 5 dotted lavender bags, 2 muted tomato bags, 4 pale fuchsia bags, 4 dim black bags.\nmirrored chartreuse bags contain 4 dark gray bags, 3 bright coral bags.\ndull black bags contain 2 dim turquoise bags, 4 drab maroon bags, 4 shiny crimson bags.\nshiny white bags contain 4 drab chartreuse bags, 4 plaid salmon bags, 1 dim green bag, 2 muted orange bags.\ndim chartreuse bags contain 3 dim bronze bags, 5 posh lavender bags, 4 drab bronze bags.\nmirrored olive bags contain 5 striped brown bags, 4 dim indigo bags.\nmuted lavender bags contain 3 dull teal bags, 4 mirrored lime bags.\nstriped teal bags contain 3 shiny coral bags.\nshiny indigo bags contain 1 dark bronze bag, 2 light lavender bags, 4 faded violet bags, 4 drab green bags.\ndim brown bags contain 5 dull aqua bags, 2 plaid indigo bags.\nlight tan bags contain 1 muted yellow bag.\ndim violet bags contain 2 dim magenta bags, 5 shiny olive bags, 1 wavy fuchsia bag, 5 dull aqua bags.\ndim crimson bags contain 2 faded bronze bags.\ndull lime bags contain no other bags.\nplaid black bags contain 2 clear beige bags, 5 faded tomato bags, 1 muted red bag.\nclear maroon bags contain 3 muted coral bags.\nfaded red bags contain 2 posh purple bags, 4 plaid gold bags, 1 bright violet bag, 3 shiny coral bags.\ndotted coral bags contain 4 pale tan bags.\ndull red bags contain 3 shiny teal bags.\nmirrored brown bags contain no other bags.\ndrab olive bags contain 2 light fuchsia bags, 1 dark brown bag, 2 shiny olive bags.\nshiny plum bags contain 3 striped olive bags, 1 mirrored brown bag, 5 faded blue bags, 4 dark bronze bags.\nplaid plum bags contain 3 shiny orange bags, 5 dim magenta bags, 2 bright crimson bags.\ndrab bronze bags contain 4 posh brown bags, 3 dotted maroon bags.\nstriped white bags contain 1 bright lime bag.\ndrab coral bags contain 1 mirrored beige bag, 4 plaid green bags, 2 drab turquoise bags, 1 drab bronze bag.\nvibrant bronze bags contain 1 muted aqua bag, 3 posh brown bags, 5 light crimson bags.\ndotted maroon bags contain 2 shiny tomato bags, 5 dark cyan bags.\nstriped plum bags contain 4 dark fuchsia bags, 4 dotted indigo bags.\nfaded indigo bags contain 4 dim orange bags, 2 vibrant crimson bags, 3 bright silver bags.\ndim magenta bags contain 1 pale red bag, 1 faded tomato bag, 3 muted aqua bags.\nmuted lime bags contain 1 wavy magenta bag.\ndrab plum bags contain 1 striped green bag.\nmirrored plum bags contain 1 bright gray bag, 4 shiny tomato bags, 1 mirrored salmon bag, 3 shiny black bags.\ndim lime bags contain 3 wavy orange bags, 1 dark orange bag, 5 vibrant indigo bags.\nfaded plum bags contain 2 shiny yellow bags, 5 dark red bags, 1 plaid bronze bag.\nshiny beige bags contain 2 striped beige bags.\nclear plum bags contain 5 vibrant violet bags, 2 vibrant silver bags, 5 dark magenta bags, 4 posh lime bags.\npale coral bags contain 1 dotted lime bag, 3 vibrant bronze bags.\ndark fuchsia bags contain 2 striped turquoise bags, 2 muted gray bags, 5 dotted turquoise bags, 2 dim black bags.\nwavy violet bags contain 5 clear fuchsia bags, 4 shiny fuchsia bags.\nwavy lime bags contain 4 plaid yellow bags, 1 striped bronze bag, 3 shiny cyan bags, 5 vibrant teal bags.\ndark coral bags contain 5 drab lime bags, 1 light brown bag, 3 pale blue bags.\nposh cyan bags contain 3 pale crimson bags, 5 wavy gray bags, 5 mirrored silver bags, 3 wavy violet bags.\nposh gold bags contain 4 plaid indigo bags, 2 mirrored fuchsia bags, 1 striped gold bag.\nlight orange bags contain 4 light coral bags, 4 shiny indigo bags.\nmirrored salmon bags contain 5 vibrant violet bags, 1 drab purple bag, 5 dark cyan bags.\nposh green bags contain 1 light crimson bag, 3 vibrant cyan bags, 2 shiny brown bags, 2 vibrant magenta bags.\nmuted gray bags contain 5 plaid chartreuse bags.\n") -> ("lines"=w1:string[])
  n2 = for {
    tunnel: w1 -> [w4] mode=indexing
    n3 = Match Pattern(string=w4, regular expression=" contain ") -> ()  [unwired: 1 in, 4 out]
  }
